vi "Stop LNA.vi"(8 "error in (no error)":errorcluster, 11 "Client Controller in":refnum<class "Client Controller.lvclass">) -> (0 "error out":errorcluster, 3 "Client Controller out":refnum<class "Client Controller.lvclass">)   [LabVIEW 2026, in "Client Controller.lvlib" / "Client Controller.lvclass"]
uses:
  Client Controller.lvclass
  Client Controller.lvclass/Client Controller.ctl
  <vilib>/ActorFramework/Message Enqueuer/Message Enqueuer.lvclass/Message Enqueuer.ctl
  <vilib>/ActorFramework/Message Enqueuer/Enqueue.vi
  <vilib>/ActorFramework/Stop Msg/Stop Msg.lvclass
  C:/Program Files/National Instruments/LabVIEW 2026/vi.lib/ActorFramework/Message/Message.lvclass
  <vilib>/ActorFramework/Message Priority Queue/Priority Enqueue.vi
  <vilib>/ActorFramework/Message Enqueuer/Message Enqueuer.lvclass
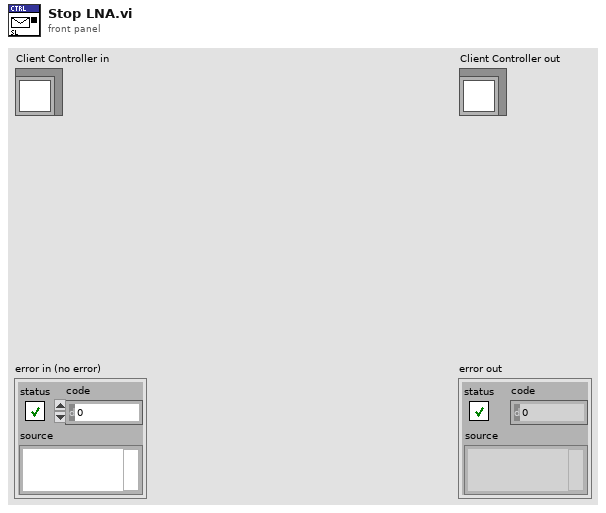
[diagram p1: front panel]
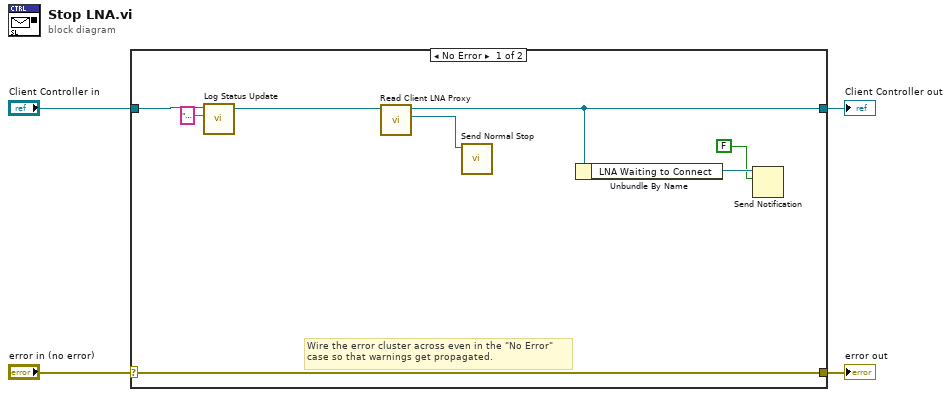
[diagram p0: block diagram]
diagram:
  n1 = case shown="No Error" "error in (no error)" {
    selector: "error in (no error)" -> [w12 w14]
    tunnel: [w12 w14] -> w3
    tunnel: [w7 w13] -> w1
    tunnel: "Client Controller in" -> [w11 w13]
    frame No Error {
      # "Wire the error cluster across even in the \"No Error\"\ncase so that warnings get propagated."
      n2 = call-dynamic "Log Status Update.vi"("String"="LNA did not connect in time.  Check that your ports are open to enable two way communication.", "Controller in"=w11) -> ("Controller out"=w9:refnum<class "Client Controller.lvclass">)  [unwired: 8 in, 1 out]
      n3 = call "Read Client LNA Proxy.vi"("Client Controller in"=w9) -> ("Actor Framework:Message Enqueuer"=w8:refnum<class "Message Enqueuer.lvclass">, "Client Controller out"=w7:refnum<class "Client Controller.lvclass">)  [unwired: 8 in, 1 out]
      n4 = call <vilib>:"Send Normal Stop.vi"("Message Enqueuer"=w8) -> ()  [unwired: 10 in, 1 out]
      n5 = Unbundle By Name(w7) -> ("LNA Waiting to Connect"=w6:refnum<notifier>)
      n6 = Send Notification(notification=FALSE, notifier=w6) -> ()  [unwired: 1 in, 2 out]
    }
    frame Error {
    }
  }
  "error out" <- w3
  "Client Controller out" <- w1
